vi "RT Loop - RSI Control.vi"(11 "Message Queue":refnum<queue>) -> ()   [LabVIEW 2018]
doc: "This RSI Control Loop VI performs control calculations on four input channels in parallel, and outputs the results to four output channels."
uses:
  support/Message Queue/Message Cluster.ctl
  <vilib>/Platform/TimedLoop/XDataNode/timing_clust.ctl
  <vilib>/Platform/TimedLoop/XDataNode/nitl_modes.ctl
  <vilib>/Platform/TimedLoop/XDataNode/wakeup.ctl
  controls/Control State.ctl
  <vilib>/Platform/TimedLoop/XDataNode/loadnilvce.vi
  <vilib>/Platform/TimedLoop/XDataNode/XDataNode.xnode
  <vilib>/Platform/TimedLoop/XDataNode/XDNodeRunTimeDep.lvlib
  support/Message Queue/Message Queue.lvlib
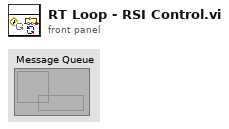
[diagram p1: front panel]
types:
  T1 = typedef "XDNodeRunTimeDep.lvlib/timing_clust.ctl" = cluster{"Expected End [f-1]":u64, "Actual End [f-1]":u64, "Finished Late? [f-1]":bool, "Expected End [i-1]":u64, "Actual End [i-1]":u64, "Finished Late? [i-1]":bool, "Expected Start [i]":u64, "Actual Start [i]":u64, "Expected Start [f]":u64, "Actual Start [f]":u64, "Source Name":string, "Structure Name":string, "Period":i64, "Deadline":i64, "Offset":i64, "Start":i64, "Priority":i32, "Timeout":i32, "Mode":T2, "Wakeup Reason":T3, "Error":errorcluster, "Source Type":string, "Secondary Source Type":string, "Global End Time":u64, "Global Start Time":u64, "Frame Duration":u64, "Iteration Duration":u64, "Assigned CPU":i32, "I/O Scan Engine Mode":u32}
  T2 = typedef "XDNodeRunTimeDep.lvlib/nitl_modes.ctl" = enum32{"No Change", "Process missed periods, maintain original phase", "Discard missed periods, maintain original phase", "Process missed periods, ignore original phase", "Discard missed periods, ignore original phase"}
  T3 = typedef "XDNodeRunTimeDep.lvlib/wakeup.ctl" = enum32{"Normal", "Aborted", "Asynchronous wakeup", "Timing source error", "Timed loop error", "Timeout"}
  T4 = typedef "Control State.ctl" = enum16{"Safe State", "Control (PID)"}
  T5 = typedef "Control Configuration.ctl" = cluster{"PID Gains":cluster{"proportional gain (Kc)":dbl, "integral gain (Kc*Ts/Ti)":dbl, "derivative gain (Kc*Td/Ts)":dbl}, "Output Range":cluster{"output high":dbl, "output low":dbl}}
  T6 = cluster{"proportional gain (Kc)":dbl, "integral gain (Kc*Ts/Ti)":dbl, "derivative gain (Kc*Td/Ts)":dbl}
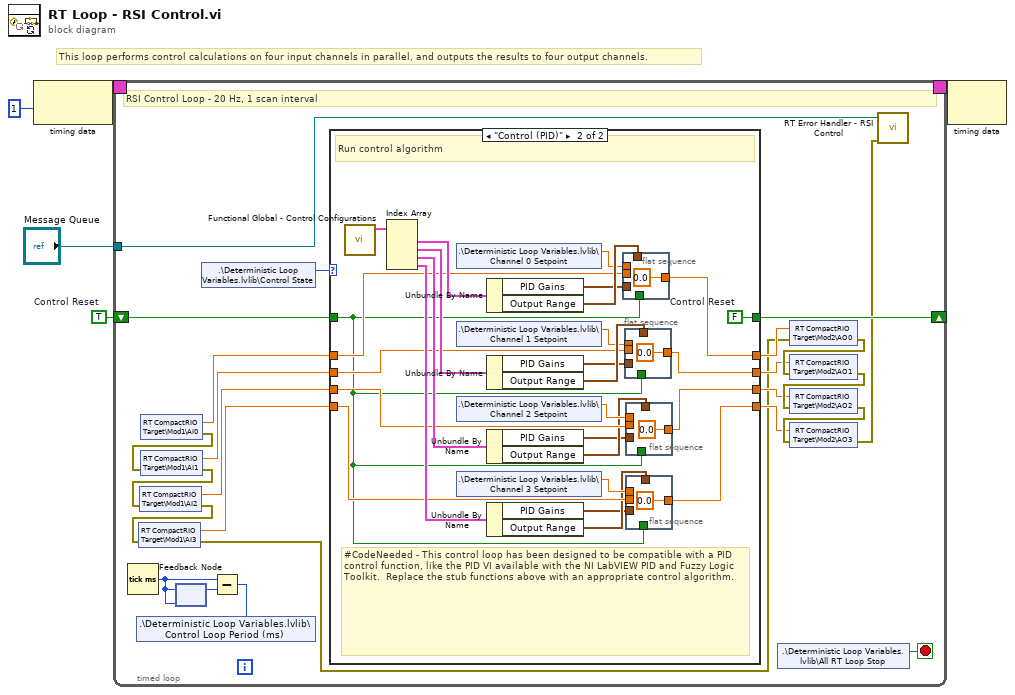
[diagram p0: block diagram]
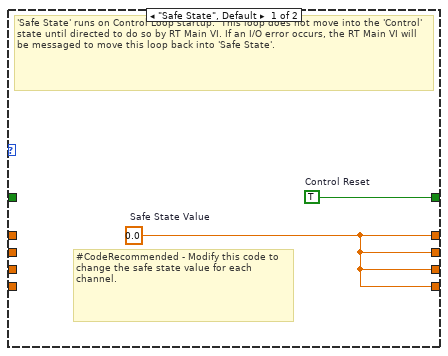
[diagram p2: hidden frame]
diagram:
  w5 = TRUE  # Control Reset
  # "This loop performs control calculations on four input channels in parallel, and outputs the results to four output channels."
  n1 = node-c288(i64 1 ("Period")) -> (w4:T1)
  n2 = timed-loop {
    shift-right: [w29] -> _
    shift-left: w5 -> [w28]
    timing: w4 -> [_]
    timing-out: [_] -> w3
    tunnel: "Message Queue" -> [w11]
    stop <- w8 stop-if-true
    # "RSI Control Loop - 20 Hz, 1 scan interval"
    n3 = Tick Count (ms)() -> (millisecond timer value=w10:u32)
    n4 = shared-variable "RT CompactRIO Target\\Mod1\\AI0"() -> (w27:dbl, error out=w26:errorcluster)  [unwired: 1 in]
    n5 = shared-variable "RT CompactRIO Target\\Mod1\\AI1"(error in=w26) -> (w23:dbl, error out=w25:errorcluster)
    n6 = shared-variable "RT CompactRIO Target\\Mod1\\AI2"(error in=w25) -> (w22:dbl, error out=w24:errorcluster)
    n7 = shared-variable "RT CompactRIO Target\\Mod1\\AI3"(error in=w24) -> (w21:dbl, error out=w13:errorcluster)
    n8 = feedback-in #1(w10) -> ()
    n9 = feedback #1(w10) -> (w9:u32)
    n10 = shared-variable ".\\Deterministic Loop Variables.lvlib\\Control State"() -> (w6:T4)  [unwired: 1 in, 1 out]
    n11 = Subtract(x=w10, y=w9) -> (x-y=w7:u32)
    n12 = shared-variable ".\\Deterministic Loop Variables.lvlib\\Control Loop Period (ms)"(w7) -> ()  [unwired: 1 in, 1 out]
    n13 = case shown="\"Control (PID)\"" w6 {
      tunnel: w27 -> [_ w49]
      tunnel: [w30 w48] -> w20
      tunnel: [w31 w58] -> w29
      tunnel: w28 -> [_ w33]
      tunnel: w23 -> [_ w44]
      tunnel: w22 -> [_ w43]
      tunnel: w21 -> [_ w37]
      tunnel: [w30 w39] -> w16
      tunnel: [w30 w38] -> w15
      tunnel: [w30 w32] -> w14
      frame "Safe State", Default {
        w30 = 0.0  # Safe State Value
        w31 = TRUE  # Control Reset
        # "#CodeRecommended - Modify this code to change the safe state value for each channel."
        # "'Safe State' runs on Control Loop startup.  This loop does not move into the 'Control' state until directed to do so by RT Main VI. If an I/O error occurs, the RT Main VI will be messaged to move this loop back into 'Safe State'."
      }
      frame "Control (PID)" {
        w58 = FALSE  # Control Reset
        # "#CodeNeeded - This control loop has been designed to be compatible with a PID control function, like the PID VI available with the NI LabVIEW PID and Fuzzy Logic Toolkit.  Replace the stub functions above with an appropriate control algorithm."
        # "Run control algorithm"
        n14 = call "Functional Global - Control Configurations.vi"() -> ("Control Configurations out"=w57:T5[])  [unwired: 11 in]
        n15 = Index Array(array=w57) -> (element #1=w56:T5, element #2=w55:T5, element #3=w54:T5, element #4=w53:T5)  [unwired: 4 in]
        n16 = shared-variable ".\\Deterministic Loop Variables.lvlib\\Channel 0 Setpoint"() -> (w50:dbl)  [unwired: 1 in, 1 out]
        n17 = shared-variable ".\\Deterministic Loop Variables.lvlib\\Channel 1 Setpoint"() -> (w45:dbl)  [unwired: 1 in, 1 out]
        n18 = shared-variable ".\\Deterministic Loop Variables.lvlib\\Channel 2 Setpoint"() -> (w42:dbl)  [unwired: 1 in, 1 out]
        n19 = shared-variable ".\\Deterministic Loop Variables.lvlib\\Channel 3 Setpoint"() -> (w36:dbl)  [unwired: 1 in, 1 out]
        n20 = Unbundle By Name(w56) -> ("PID Gains"=w51:T6, "Output Range"=w52:cluster{"output high":dbl, "output low":dbl})
        n21 = Unbundle By Name(w55) -> ("PID Gains"=w46:T6, "Output Range"=w47:cluster{"output high":dbl, "output low":dbl})
        n22 = Unbundle By Name(w54) -> ("PID Gains"=w40:T6, "Output Range"=w41:cluster{"output high":dbl, "output low":dbl})
        n23 = Unbundle By Name(w53) -> ("PID Gains"=w34:T6, "Output Range"=w35:cluster{"output high":dbl, "output low":dbl})
        n24 = flat-sequence {
          tunnel: w52 -> [_]
          tunnel: w51 -> [_]
          tunnel: w50 -> [_]
          tunnel: w49 -> [_]
          tunnel: [0.0 ("Safe State Value")] -> w48
          tunnel: w33 -> [_]
          frame #0 {
          }
        }
        n25 = flat-sequence {
          tunnel: w47 -> [_]
          tunnel: w46 -> [_]
          tunnel: w45 -> [_]
          tunnel: w44 -> [_]
          tunnel: [0.0 ("Safe State Value")] -> w39
          tunnel: w33 -> [_]
          frame #0 {
          }
        }
        n26 = flat-sequence {
          tunnel: w43 -> [_]
          tunnel: w42 -> [_]
          tunnel: w41 -> [_]
          tunnel: w40 -> [_]
          tunnel: [0.0 ("Safe State Value")] -> w38
          tunnel: w33 -> [_]
          frame #0 {
          }
        }
        n27 = flat-sequence {
          tunnel: w37 -> [_]
          tunnel: w36 -> [_]
          tunnel: w35 -> [_]
          tunnel: w34 -> [_]
          tunnel: w33 -> [_]
          tunnel: [0.0 ("Safe State Value")] -> w32
          frame #0 {
          }
        }
      }
    }
    n28 = shared-variable ".\\Deterministic Loop Variables.lvlib\\All RT Loop Stop"() -> (w8:bool)  [unwired: 1 in, 1 out]
    n29 = shared-variable "RT CompactRIO Target\\Mod2\\AO0"(w20, error in=w13) -> (error out=w19:errorcluster)
    n30 = shared-variable "RT CompactRIO Target\\Mod2\\AO1"(w16, error in=w19) -> (error out=w18:errorcluster)
    n31 = shared-variable "RT CompactRIO Target\\Mod2\\AO2"(w15, error in=w18) -> (error out=w17:errorcluster)
    n32 = shared-variable "RT CompactRIO Target\\Mod2\\AO3"(w14, error in=w17) -> (error out=w12:errorcluster)
    n33 = call "RT Error Handler - RSI Control.vi"("error in (no error)"=w12, "Message Queue"=w11) -> ()  [unwired: 8 in, 2 out]
  }
  n34 = node-c288(w3) -> ()  [unwired: 1 out]
